vi "SetCommandStatus_GIS Printer.vi"(8 "error in (no error)":errorcluster, 9 "Command Data":T1, 10 "Command":string, 11 "GIS Printer In":refnum<class "GIS Printer.lvclass">) -> (0 "error out":errorcluster, 3 "GIS Printer Out":refnum<class "GIS Printer.lvclass">)   [LabVIEW 2022 SP3, in "GIS Printer.lvclass"]
uses:
  GIS Printer.lvclass
  Typedefs/Command Data.ctl
  Typedefs/PrinterCmdStatus--Enum.ctl
  GIS Printer.lvclass/GIS Printer.ctl
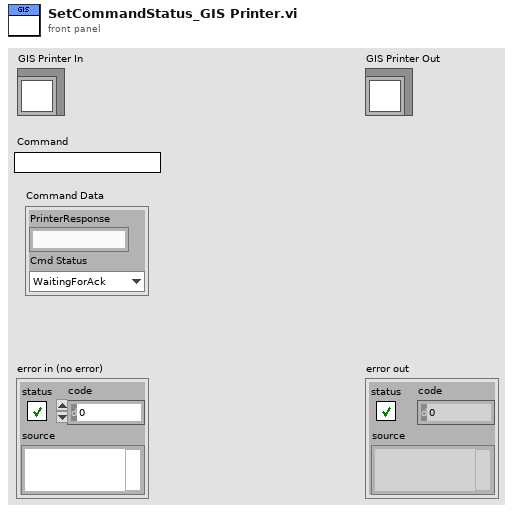
[diagram p1: front panel]
types:
  T1 = typedef "GIS Printer.lvclass/Command Data.ctl" = cluster{"PrinterResponse":string, "Cmd Status":T2}
  T2 = typedef "GIS Printer.lvclass/PrinterCmdStatus--Enum.ctl" = enum16{"WaitingForAck", "Executing", "Executing Standby", "Completed", "Error"}
  T3 = typedef "GIS Printer.lvclass/Private Data.ctl" = cluster{"UserEvents":T4, "All Dependencies":cluster{"Class References":refnum<class>[], "Class Names":string[]}, "PrinterConiguration":T5, "Status":T6}
  T4 = typedef "GIS Printer.lvclass/UserEvents.ctl" = cluster{"API Incoming Event":refnum<user-event>, "API Executed Event":refnum<user-event>, "API Return Event":refnum<user-event>, "Status Changed Event":refnum<user-event>, "Abort":refnum<user-event>, "stop process":refnum<user-event>}
  T5 = typedef "GIS Printer.lvclass/PrinterConfiguration--Cluster.ctl" = cluster{"IPAddress":string, "Move Stage on RTP Command?":bool, "Stage Move Position":string, "PH1-Prime Path":path, "PH2-Prime Path":path, "PH3-Prime Path":path, "PH4-Prime Path":path, "PH5-Prime Path":path, "PH6-Prime Path":path, "PrintScriptsFolder":path, "PurgeScriptsFolder":path, "StageScriptsFolder":path, "PH1-HeatOn Path":path, "PH2-HeatOn Path":path, "PH3-HeatOn Path":path, "PH4-HeatOn Path":path, "PH5-HeatOn Path":path, "PH6-HeatOn Path":path, "PH1-HeatOff Path":path, "PH2-HeatOff Path":path, "PH3-HeatOff Path":path, "PH4-HeatOff Path":path, "PH5-HeatOff Path":path, "PH6-HeatOff Path":path}
  T6 = typedef "GIS Printer.lvclass/Status Cluster.ctl" = cluster{"Command Status":variant, "TCP Commands & Responses":string[][], "Printer Busy?":bool}
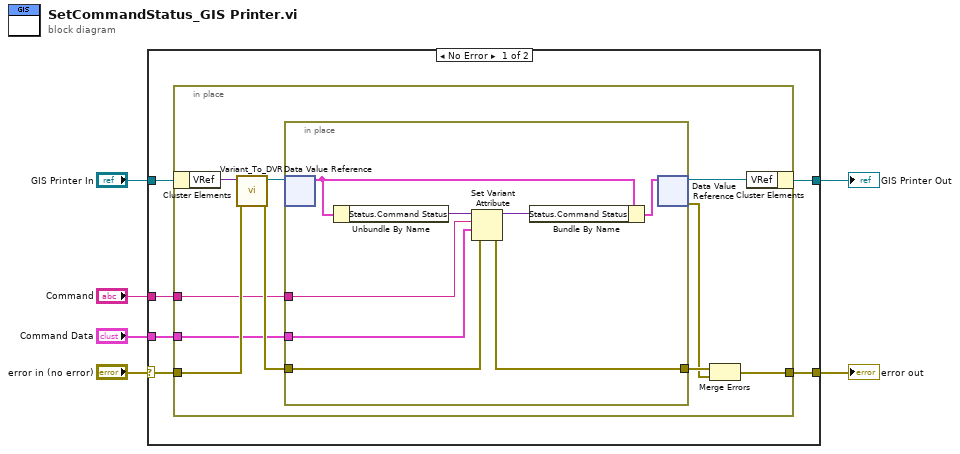
[diagram p0: block diagram]
diagram:
  n1 = case shown="No Error" "error in (no error)" {
    selector: "error in (no error)" -> [w9 w32]
    tunnel: [w11 w32] -> w5
    tunnel: [w12 w31] -> w3
    tunnel: "GIS Printer In" -> [w10 w31]
    tunnel: "Command" -> [w8 _]
    tunnel: "Command Data" -> [w7 _]
    frame No Error {
      n2 = in-place {
        in-place-border: w9 -> [w20]
        in-place-border: [w16] -> w11
        in-place-border: w8 -> [w14]
        in-place-border: w7 -> [w13]
        n3 = in-place-cluster #1(w10) -> ("VRef"=w22:variant)
        n4 = call "Variant_To_DVR.vi"("error in (no error)"=w20, "Variant"=w22) -> ("error out"=w19:errorcluster, "DVR"=w21:refnum<data-value>)  [unwired: 8 in]
        n5 = in-place {
          in-place-border: w19 -> [w25]
          in-place-border: [w26] -> w18
          in-place-border: w14 -> [w24]
          in-place-border: w13 -> [w23]
          n6 = in-place-dvr #2(w21) -> (w29:T3)  [unwired: 1 out]
          n7 = Unbundle By Name(w29) -> ("Status.Command Status"=w30:variant)
          n8 = Set Variant Attribute(Variant=w30, name=w24, value=w23, error in=w25) -> (Variant out=w28:variant, error out=w26:errorcluster)  [unwired: 1 out]
          n9 = Bundle By Name(cluster=w29, "Status.Command Status"=w28) -> (w27:T3)
          n10 = in-place-dvr #2(w27) -> (w15:refnum<data-value>, w17:errorcluster)
        }
        n11 = Merge Errors(w18, w17) -> (w16:errorcluster)
        n12 = in-place-cluster #1("VRef"=w15) -> (w12:refnum<class "GIS Printer.lvclass">)
      }
    }
    frame Error {
    }
  }
  "error out" <- w5
  "GIS Printer Out" <- w3
